vi "Scroll-Vmove.vi"(8 "error in (no error)":errorcluster, 9 "New coordinate":T1, 11 "Gviewer in":refnum<class "Gviewer.lvclass">) -> (0 "error out":errorcluster, 1 "delta V":i32, 3 "Gviewer out":refnum<class "Gviewer.lvclass">)   [LabVIEW 2020, in "Sgraph_lib_V1.lvlib" / "Gviewer.lvclass"]
doc: "Andre Koelewijn, 31 jan 2021\n\nThis VI perform the actual vertical move in respect to the position where the mouse was clicked."
uses:
  Gviewer.lvclass
  <vilib>/Utility/miscctls.llb/LVPoint32TypeDef.ctl
  Gviewer.lvclass/Gviewer.ctl
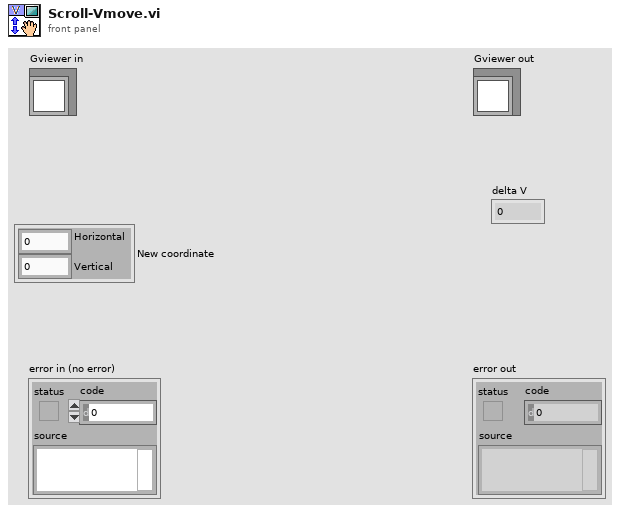
[diagram p1: front panel]
types:
  T1 = typedef "LVPoint32TypeDef.ctl" = cluster{"Horizontal":i32, "Vertical":i32}
  T2 = typedef "Sgraph_lib_V1.lvlib/Gviewer.lvclass/Typedef_SelProperties.ctl" = cluster{"Color":u32, "LineType":T3, "max":dbl, "min":dbl}
  T3 = typedef "Sgraph_lib_V1.lvlib/Gviewer.lvclass/Typedef_LineType.ctl" = enum16{"num_bare", "num_MinMax_Area", "num_MinMax_Lines", "num_MinMax_Forfor", "num_Max_Area", "num_Max_Line", "num_Max_Forfor", "num_Min_Area", "num_Min_Line", "num_Min_Fosfor", "Boolean_Line_01", "Boolean_Area_01", "Boolean_Fosfor_01", "Boolean_Line_TF", "Boolean_Area_TF", "Boolean_Fosfor_TF", "Boolean_OnOff_Line", "Boolean_OnOff_Area", "Boolean_OnOff_Fosfor", "Boolean_spare", "StringEvent_Line", "StringEvent_TimeLine"}
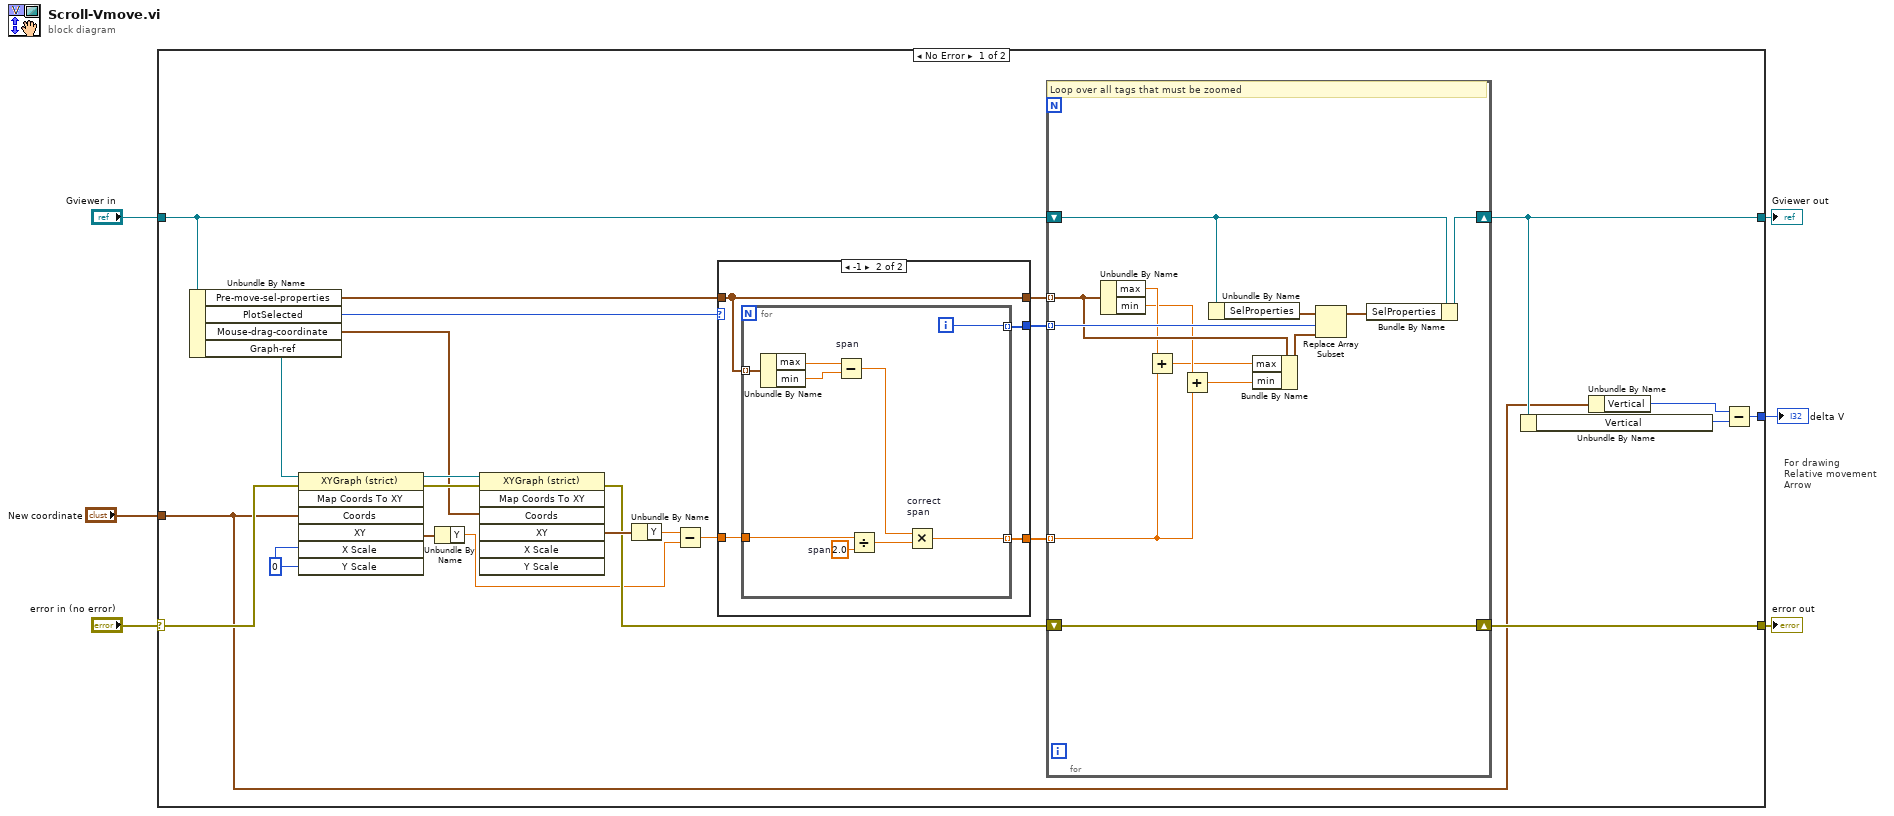
[diagram p0: block diagram]
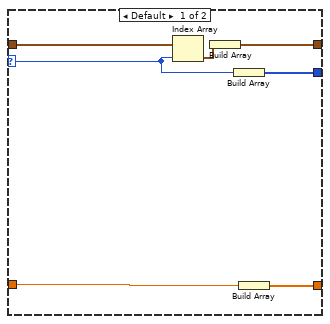
[diagram p2: hidden frame]
diagram:
  # "For drawing\nRelative movement\nArrow"
  n1 = case shown="No Error" "error in (no error)" {
    selector: "error in (no error)" -> [w23 w65]
    tunnel: [w28 w65] -> w5
    tunnel: [w18 w64] -> w3
    tunnel: "Gviewer in" -> [w22 w64]
    tunnel: "New coordinate" -> [w17 _]
    tunnel: [w19 _] -> w1
    frame No Error {
      w26 = 0 ("Y Scale")
      n2 = Unbundle By Name(w22) -> ("Pre-move-sel-properties"=w29:T2[], "PlotSelected"=w30:i32, "Mouse-drag-coordinate"=w12:T1, "Graph-ref"=w11:refnum<vi>)
      n3 = invoke class="XYGraph (strict)" method="Map Coords To XY"(reference=w11, error in=w23, "Coords"=w17, "X Scale"=w26, "Y Scale"=w26) -> (reference out=w14:refnum<vi>, error out=w15:errorcluster, "XY"=w25:cluster{"X":dbl, "Y":dbl})  [unwired: 2 in, 4 out]
      n4 = Unbundle By Name(w25) -> ("Y"=w8:dbl)
      n5 = invoke class="XYGraph (strict)" method="Map Coords To XY"(reference=w14, error in=w15, "Coords"=w12) -> (error out=w13:errorcluster, "XY"=w16:cluster{"X":dbl, "Y":dbl})  [unwired: 4 in, 5 out]
      n6 = Unbundle By Name(w16) -> ("Y"=w9:dbl)
      n7 = Subtract(x=w9, y=w8) -> (x-y=w7:dbl)
      n8 = case shown="-1" w30 {
        selector: w30 -> [w47 _]
        tunnel: w29 -> [w49 w53]
        tunnel: [w50 w53] -> w27
        tunnel: [w46 w54] -> w24
        tunnel: [w45 w52] -> w10
        tunnel: w7 -> [w44 w51]
        frame Default {
          n9 = Index Array(array=w49, index=w47) -> (element=w48:T2)
          n10 = Build Array(w48) -> (w50:T2[])
          n11 = Build Array(w47) -> (w46:i32[])
          n12 = Build Array(w44) -> (w45:dbl[])
        }
        frame -1 {
          n13 = for {
            tunnel: [w63] -> w54 mode=indexing
            tunnel: w53 -> [w57] mode=indexing
            tunnel: [w56] -> w52 mode=indexing
            tunnel: w51 -> [w55]
            i -> [w63]
            w58 = 2.0  # span
            n14 = Unbundle By Name(w57) -> ("max"=w62:dbl, "min"=w59:dbl)
            n15 = Subtract "span"(x=w62, y=w59) -> (x-y=w60:dbl)
            n16 = Divide(x=w55, y=w58) -> (x/y=w61:dbl)
            n17 = Multiply "correct\nspan"(x=w60, y=w61) -> (x*y=w56:dbl)
          }
        }
      }
      n18 = for {
        shift-right: [w31] -> w18
        shift-left: w22 -> [w32]
        shift-right: [w43] -> w28
        shift-left: w13 -> [w43]
        tunnel: w27 -> [w39] mode=indexing
        tunnel: w24 -> [w40] mode=indexing
        tunnel: w10 -> [w33] mode=indexing
        # "Loop over all tags that must be zoomed"
        n19 = Unbundle By Name(w39) -> ("max"=w37:dbl, "min"=w36:dbl)
        n20 = Add(x=w37, y=w33) -> (x+y=w35:dbl)
        n21 = Add(x=w36, y=w33) -> (x+y=w34:dbl)
        n22 = Unbundle By Name(w32) -> ("SelProperties"=w42:T2[])
        n23 = Bundle By Name(cluster=w39, "max"=w35, "min"=w34) -> (w38:T2)
        n24 = Replace Array Subset(array=w42, new element=w38, index=w40) -> (w41:T2[])
        n25 = Bundle By Name(cluster=w32, "SelProperties"=w41) -> (w31:refnum<class "Gviewer.lvclass">)
      }
      n26 = Unbundle By Name(w18) -> ("Vertical"=w21:i32)
      n27 = Unbundle By Name(w17) -> ("Vertical"=w20:i32)
      n28 = Subtract(x=w20, y=w21) -> (x-y=w19:i32)
    }
    frame Error {
    }
  }
  "error out" <- w5
  "Gviewer out" <- w3
  "delta V" <- w1
